vi "Linear Fit (LAR).vi"(0 "Y":dbl[](array[numeric]) format="%#.6g", 5 "X":dbl[](array[numeric]) format="%#.6g", 7 "Weight":dbl[](array[numeric]) format="%#.6g", 9 "tol":dbl=0.0001) -> (4 "Best Linear Fit":dbl[](array[numeric]) format="%#.6g", 6 "slope":dbl format="%#.6g", 8 "intercept":dbl format="%#.6g", 14 "residue":dbl format="%#.6g", 15 "error":i32)   [LabVIEW 2017, in "NI_AALPro.lvlib"]
uses:
  <vilib>/Analysis/NI_AALPro.lvlib
  <resource>/lvanlys.dll
panel:
  # "LAR Linear Fit"
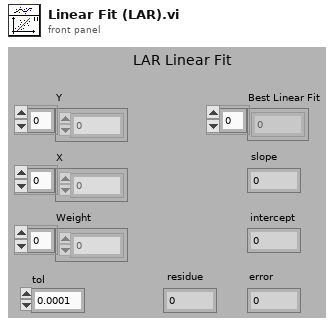
[diagram p1: front panel]
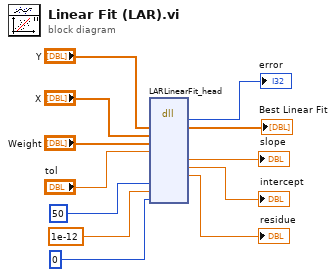
[diagram p0: block diagram]
diagram:
  n1 = dll-call lib="e:/builds/penguin/labview/branches/2017/dev/dist/resource/lvanlys.*" fn="LARLinearFit_head"("yH"="Y", "xH"="X", "weight"="Weight", "tol"="tol", "maxIter"=50, "absTol"=1e-12, "isCoef"=0) -> (→"error":i32, "yH"=→"Best Linear Fit":dbl[], "slope"=→"slope":dbl, "intercept"=→"intercept":dbl, "meanErr"=→"residue":dbl)  [unwired: 12 in, 2 out]
